vi "FPGA_SICK Read Response.vi"(8 "error in (no error)":errorcluster, 9 "Timeout (ms)":i32, 11 "Response Index":u32) -> (0 "error out":errorcluster, 1 "Timed Out":bool, 2 "Current response length":u8, 3 "Correct Response Read?":bool)   [LabVIEW 2009]
uses:
  <vilib>/rvi/DataTransferAndStorage/Container/XNode/niFpgaContainer.xnode
  <vilib>/rvi/Memory/Memory_Emulation/nirvimemoryEmulationManagerCache_GetValue.vi
  <vilib>/rvi/Memory/Memory_Emulation/nirvimemoryEmulationManagerCache_InsertValue.vi
  <vilib>/rvi/DataTransferAndStorage/Container/Common/niFpgaContainerGetUniqueNameForEmu.vi
  <vilib>/Utility/error.llb/Clear Errors.vi
  <vilib>/rvi/Memory/Memory_Emulation/nirvimemoryEmulationManagerCache_SetValue.vi
  <vilib>/eio/EIOMethodNode/EIOMethodNode.xnode
  <vilib>/rvi/eio/nirviEIOMethodImplementation/nirviEIOMethodImplementation.xnode
  <vilib>/rvi/eio/common/nirviEmuTemplateMethod_errors.vi
  <vilib>/rvi/eio/common/nirviEmuClasses.ctl
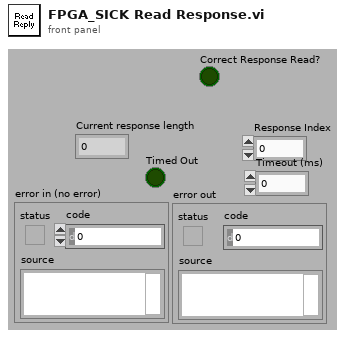
[diagram p1: front panel]
types:
  T1 = typedef "nirviEmuClasses.ctl" = enum16{"IO Read", "IO Write", "Method", "Property Read", "Property Write"}
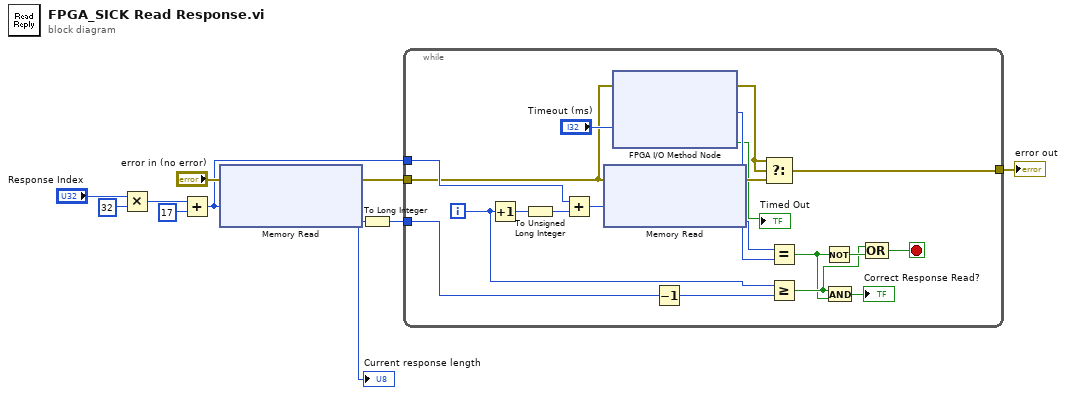
[diagram p0: block diagram]
diagram:
  n1 = Multiply(x="Response Index", y=u32 32) -> (x*y=w9:u32)
  n2 = Add(x=w9, y=u32 17) -> (x+y=w3:u32)
  n3 = xnode ("Memory Read")("Address"=w3, "error in (no error)"="error in (no error)") -> ("Data"=w7:u8, "error out"=w4:errorcluster)  [unwired: 1 in, 1 out]
  "Current response length" <- w7
  n4 = To Long Integer(number=w7) -> (32bit integer=w6:i32)
  n5 = while {
    tunnel: w3 -> [w30]
    tunnel: w6 -> [w26]
    tunnel: w4 -> [w18]
    tunnel: [w15] -> w1
    i -> [w20]
    stop <- w24 stop-if-true
    n6 = Increment(x=w20) -> (x+1=w28:i32)
    n7 = To Unsigned Long Integer(number=w28) -> (unsigned 32bit integer=w29:u32)
    n8 = Add(x=w30, y=w29) -> (x+y=w27:u32)
    n9 = xnode ("Memory Read")("Address"=w27, "error in (no error)"=w18) -> ("Data"=w23:u8, "error out"=w16:errorcluster)  [unwired: 1 in, 1 out]
    n10 = xnode "FPGA I/O Method Node"("error in"=w18, "Timeout (ms)"="Timeout (ms)") -> ("error out"=w17:errorcluster, "Data"=w22:u8, "Timed Out"=→"Timed Out":bool)  [unwired: 1 in, 1 out]
    n11 = Decrement(x=w26) -> (x-1=w25:i32)
    n12 = Select(t=w17, s=w17, f=w16) -> (s? t:f=w15:errorcluster)
    n13 = Equal?(x=w23, y=w22) -> (x = y?=w13:bool)
    n14 = Greater Or Equal?(x=w20, y=w25) -> (x >= y?=w14:bool)
    n15 = Not(x=w13) -> (.not. x?=w21:bool)
    n16 = And(x=w14, y=w13) -> (x .and. y?=→"Correct Response Read?":bool)
    n17 = Compound Arithmetic op=OR(w14, w21) -> (w24:bool)
  }
  "error out" <- w1
